vi "p2.vi"() -> ()   [LabVIEW 2021, in "d14.lvlib"]
uses:
  d14.lvlib
  AOC/AOC.lvlib
panel:
  out "XY Graph":cluster{"Left out":u32[], "Top out":u32[]}[](graph)
  in  "Example":string="498,4 -> 498,6 -> 496,6\n503,4 -> 502,4 -> 502,9 -> 494,9"
  in  "Example":bool
  out "Answer":i64
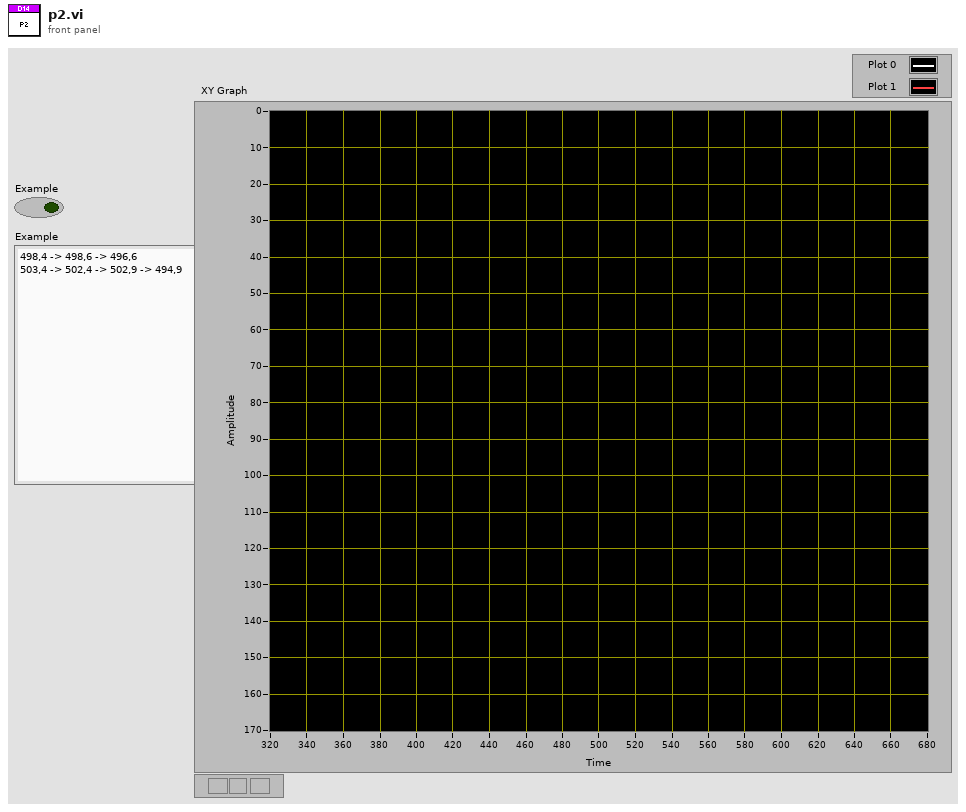
[diagram p1: front panel]
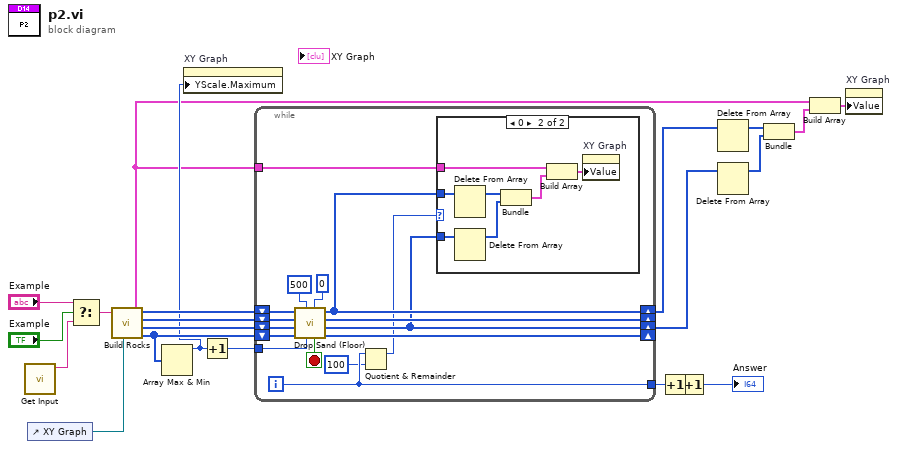
[diagram p0: block diagram]
diagram:
  n1 = call "Get Input.vi"() -> ("Input"=w21:string)  [unwired: 11 in]
  n2 = control-ref of="XY Graph"() -> (w11:refnum<vi>)
  n3 = Select(t="Example", s="Example", f=w21) -> (s? t:f=w15:string)
  n4 = call "Build Rocks.vi"("reference"=w11, "Input"=w15) -> ("Bottom"=w14:i32[], "Top"=w17:i32[], "Right"=w16:i32[], "Left"=w18:i32[], "Rocks"=w2:cluster{u32[], u32[]})  [unwired: 4 in, 1 out]
  n5 = Array Max & Min(array=w14) -> (max value=w10:i32)  [unwired: 3 out]
  n6 = property on="XY Graph" class="XYGraph (strict)"("YScale.Maximum"=w10) -> ()  [unwired: 2 in, 2 out]
  n7 = Increment(x=w10) -> (x+1=w13:i32)
  n8 = while {
    tunnel: [w27] -> w12
    shift-right: [w24] -> w3
    shift-left: w18 -> [w36]
    shift-right: [w30] -> _
    shift-left: w16 -> [w35]
    shift-right: [w23] -> w8
    shift-left: w17 -> [w37]
    shift-right: [w29] -> _
    shift-left: w14 -> [w34]
    tunnel: w13 -> [w28]
    tunnel: w2 -> [w25]
    i -> [w27]
    stop <- w33 stop-if-true
    n9 = call "Drop Sand (Floor).vi"("Y in"=0, "Floor-1"=w28, "X in"=500, "Bottom in"=w34, "Top in"=w37, "Right in"=w35, "Left in"=w36) -> ("Bottom out"=w29:i32[], "Top out"=w23:i32[], "Right out"=w30:i32[], "Left out"=w24:i32[], "Filled?"=w33:bool)
    n10 = Quotient & Remainder(x=w27, y=100) -> (x-y*floor(x/y)=w22:i32)  [unwired: 1 out]
    n11 = case shown="0" w22 {
      tunnel: w25 -> [_ w44]
      tunnel: w24 -> [_ w41]
      tunnel: w23 -> [_ w39]
      frame Default {
      }
      frame 0 {
        n12 = Delete From Array(array=w41) -> (array with subset deleted=w40:i32[])  [unwired: 2 in, 1 out]
        n13 = Delete From Array(array=w39) -> (array with subset deleted=w38:i32[])  [unwired: 2 in, 1 out]
        n14 = Bundle("Left out"=w40, "Top out"=w38) -> (w42:cluster{"Left out":i32[], "Top out":i32[]})  [unwired: 1 in]
        n15 = Build Array(w44, w42) -> (w43:cluster{"Left out":u32[], "Top out":u32[]}[])
        n16 = property on="XY Graph" class="XYGraph (strict)"("Value"=w43) -> ()  [unwired: 2 in, 2 out]
      }
    }
  }
  n17 = Increment(x=w12) -> (x+1=w9:i32)
  n18 = Increment(x=w9) -> (x+1=→"Answer":i32)
  n19 = Delete From Array(array=w3) -> (array with subset deleted=w5:i32[])  [unwired: 2 in, 1 out]
  n20 = Delete From Array(array=w8) -> (array with subset deleted=w4:i32[])  [unwired: 2 in, 1 out]
  n21 = Bundle("Left"=w5, "Top"=w4) -> (w6:cluster{"Left":i32[], "Top":i32[]})  [unwired: 1 in]
  n22 = Build Array(w2, w6) -> (w7:cluster{"Left":u32[], "Top":u32[]}[])
  n23 = property on="XY Graph" class="XYGraph (strict)"("Value"=w7) -> ()  [unwired: 2 in, 2 out]
